vi "test.cfgTable.vi"() -> ()   [LabVIEW 2017]
uses:
  0ce3606b-4a8d-450a-b335-de3da5102bc9.vi
  baa86c02-3178-42a1-8f26-a93653cd2720.vi
  Configuration/ClusterCfgTable/Flatten Cluster To CfgTable.vi
  Configuration/ClusterCfgTable/Parse CfgTable.vi
panel:
  out "error out":errorcluster
  out "Cluster Configuration Out":cluster{dbl[unit]}
  out "CfgTable Row":string[](array[string])
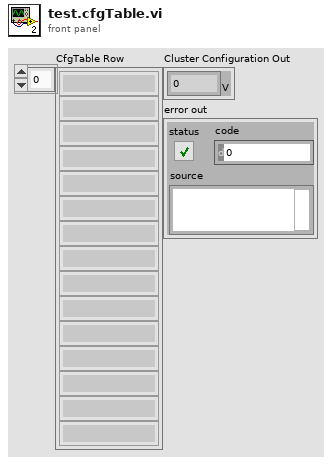
[diagram p1: front panel]
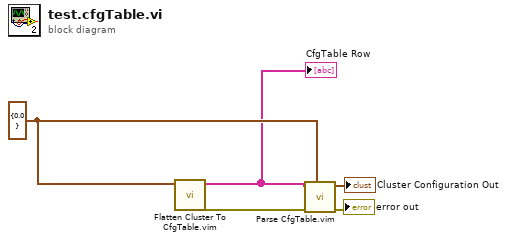
[diagram p0: block diagram]
diagram:
  w5 = cluster{dbl[unit]} {0.0}
  n1 = call "Flatten Cluster To CfgTable.vim"("Cluster Configuration Typedef"=w5) -> ("error out"=w2:errorcluster, "CfgTable Row"=w4:string[])  [unwired: 9 in]
  "CfgTable Row" <- w4
  n2 = call "Parse CfgTable.vim"("Cluster Configuration Typedef"=w5, "error in (no error)"=w2, "CfgTable Row"=w4) -> ("error out"=→"error out":errorcluster, "Cluster Configuration Out"=→"Cluster Configuration Out":cluster{dbl[unit]})  [unwired: 7 in]
